vi "DiscreteDerivative_subsubsubvi.vi"(10 "data":dbl, 11 "deltaT":dbl) -> (3 "(data-data_old)/delT":dbl)   [LabVIEW 2019]
panel:
  out "data_old":dbl
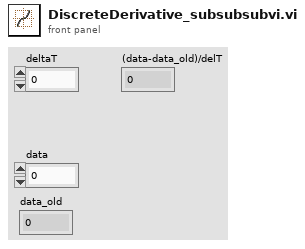
[diagram p1: front panel]
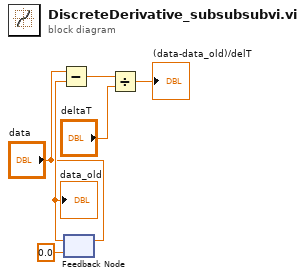
[diagram p0: block diagram]
diagram:
  n1 = feedback #1(0.0 ("data")) -> (w4:dbl)
  "data_old" <- w4
  n2 = Subtract(x="data", y=w4) -> (x-y=w5:dbl)
  n3 = feedback-in #1("data") -> ()
  n4 = Divide(x=w5, y="deltaT") -> (x/y=→"(data-data_old)/delT":dbl)
